vi "NeoceraLoadCalibration.vi"() -> ()   [LabVIEW 2012]
panel:
  in  "Neocera name":refnum<visa-resource-name>
  in  "Calibration file path":path
  in  "Resistance column":i32=1
  in  "Temperature column":i32
  in  "Sort temperature":bool=TRUE
  out "data string":string="$;"
  out "?":string="SCALT4,2,1,x08257,-1,"
  out "?":string="300.000000,34.000000,"
  out "?":T1(graph)
  in  "Multiplier":dbl=-1.0
  in  "Sensor description":string
  in  "Calibration table units":u16(ring)=1 items=["Log Ohms", "Ohms", "Volts"]
  in  "AC Voltage Bias":u16(ring)=2 items=["10mV", "3mV", "1mV", "320uV", "100uV", "32uV", "10uV"]
  in  "Sensor type":u16(ring)=4 items=["2V Diode", "6V Diode", "Ohms DC 1mA", "Ohms DC 10uA", "Ohms AC"]
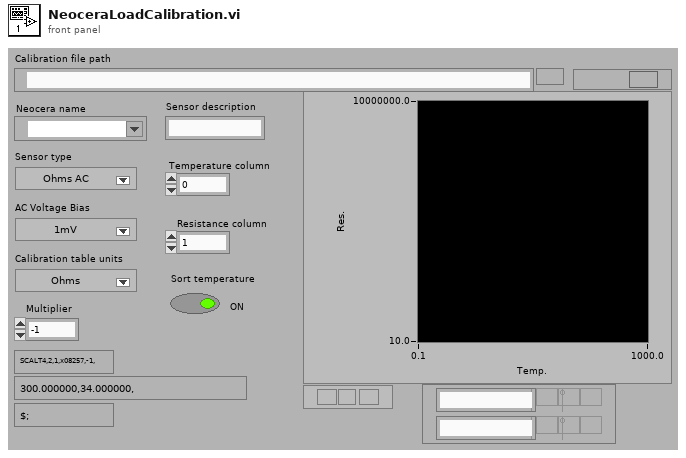
[diagram p1: front panel]
types:
  T1 = cluster{"Sorted Array":dbl[], "Sorted Array":dbl[]}
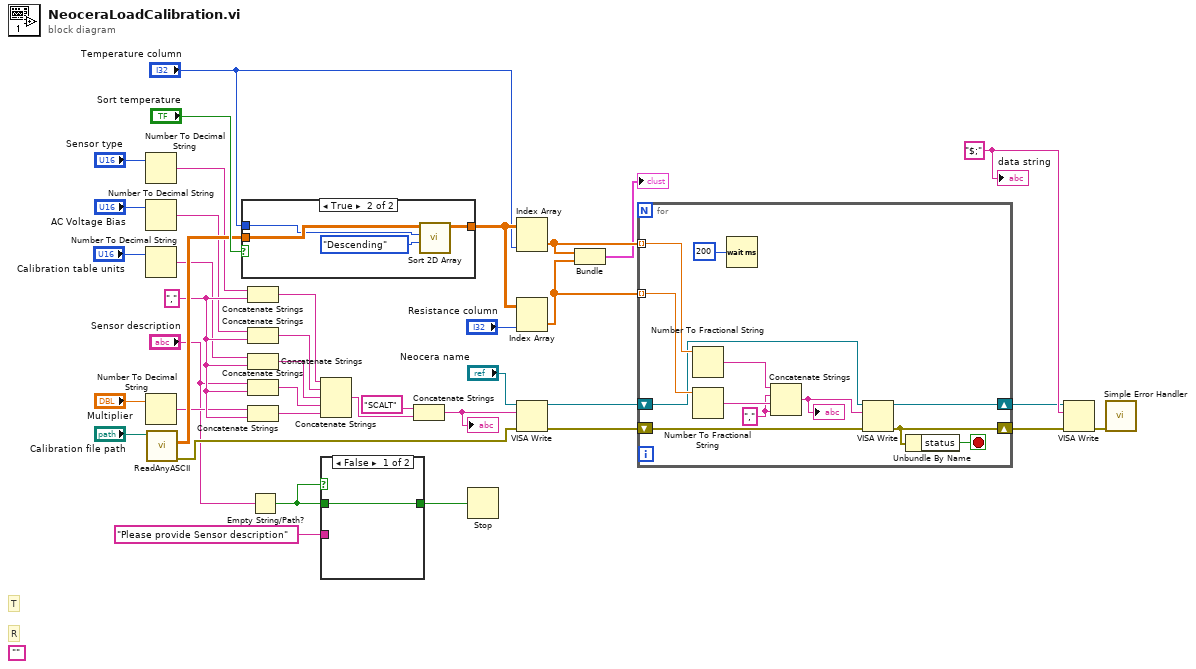
[diagram p0: block diagram]
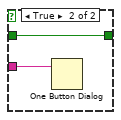
[diagram p2: hidden frame]
diagram:
  w22 = ","
  w36 = "$;"
  (unwired) ""
  # "R"
  # "T"
  n1 = Number To Decimal String(number="Sensor type") -> (decimal integer string=w20:string)  [unwired: 1 out]
  n2 = Number To Decimal String(number="AC Voltage Bias") -> (decimal integer string=w16:string)  [unwired: 1 out]
  n3 = Number To Decimal String(number="Calibration table units") -> (decimal integer string=w15:string)  [unwired: 1 out]
  n4 = Number To Decimal String(number="Multiplier") -> (decimal integer string=w14:string)  [unwired: 1 out]
  n5 = call "ReadAnyASCII.vi"("file path (dialog if empty)"="Calibration file path") -> ("error out"=w23:errorcluster, "all rows"=w27:dbl[][])  [unwired: 3 in, 6 out]
  n6 = case shown="True" "Sort temperature" {
    tunnel: w27 -> [w39 w43]
    tunnel: [w39 w41] -> w26
    tunnel: "Temperature column" -> [_ w42]
    frame False {
    }
    frame True {
      n7 = call "Sort 2D Array.vi"("Order"=enum16{"Ascending", "Descending"}."Descending", "Sort column #"=w42, "Array"=w43) -> ("Sorted Array"=w41:dbl[][])  [unwired: 4 out]
    }
  }
  n8 = Concatenate Strings(w20, w22) -> (w13:string)
  n9 = Concatenate Strings(w16, w22) -> (w12:string)
  n10 = Concatenate Strings(w15, w22) -> (w11:string)
  n11 = Concatenate Strings("Sensor description", w22) -> (w10:string)
  n12 = Concatenate Strings(w14, w22) -> (w9:string)
  n13 = Empty String/Path?(string/path="Sensor description") -> (empty?=w6:bool)
  n14 = Concatenate Strings(w13, w12, w11, w10, w9) -> (w32:string)
  n15 = case shown="False" w6 {
    tunnel: "Please provide Sensor description" ("message") -> [_ w46]
    tunnel: w6 -> [w44 w45]
    tunnel: [w44 w45] -> w5
    frame False {
    }
    frame True {
      n16 = One Button Dialog(message=w46) -> ()  [unwired: 2 out]
    }
  }
  n17 = Concatenate Strings("SCALT" ("data string"), w32) -> (w33:string)
  "?" <- w33
  n18 = Stop(stop? (T)=w5) -> ()
  n19 = Index Array(array=w26, index (col)="Temperature column") -> (element=w37:dbl[])  [unwired: 1 in]
  n20 = Index Array(array=w26, index (col)="Resistance column") -> (element=w38:dbl[])  [unwired: 1 in]
  n21 = VISA Write(VISA resource name="Neocera name", write buffer=w33, error in (no error)=w23) -> (VISA resource name out=w1:refnum<visa-resource-name>, error out=w3:errorcluster)  [unwired: 1 out]
  n22 = Bundle("Sorted Array"=w37, "Sorted Array"=w38) -> (→"?":T1)  [unwired: 1 out]
  n23 = for {
    tunnel: w38 -> [w55] mode=indexing
    tunnel: w37 -> [w56] mode=indexing
    shift-right: [w53] -> w35
    shift-left: w3 -> [w54]
    shift-right: [w47] -> w4
    shift-left: w1 -> [w48]
    stop <- w52 stop-if-true
    w50 = ","
    n24 = Number To Fractional String(number=w56) -> (F-format string=w58:string)  [unwired: 3 out]
    n25 = Number To Fractional String(number=w55) -> (F-format string=w51:string)  [unwired: 3 out]
    n26 = Wait (ms)(milliseconds to wait=u32 200) -> ()  [unwired: 1 out]
    n27 = Concatenate Strings(w58, w50, w51, w50) -> (w49:string)
    "?" <- w49
    n28 = VISA Write(VISA resource name=w48, write buffer=w49, error in (no error)=w54) -> (VISA resource name out=w47:refnum<visa-resource-name>, error out=w53:errorcluster)  [unwired: 1 out]
    n29 = Unbundle By Name(w53) -> ("status"=w52:bool)
  }
  n30 = VISA Write(VISA resource name=w4, write buffer=w36, error in (no error)=w35) -> (error out=w34:errorcluster)  [unwired: 2 out]
  n31 = call <vilib>:"Simple Error Handler.vi"("error in (no error)"=w34) -> ()  [unwired: 1 in, 8 out]
  "data string" <- w36
